vi "ConfigureElevator.vi"(10 "Talon In":T1) -> (2 "Talon Out":T1)   [LabVIEW 2018]
uses:
  <vilib>/Rock Robotics/WPI/MotorControl/WPI_MotorControlDeviceRef.ctl
  <vilib>/Rock Robotics/WPI/MotorControl/WPI_MotorControlType.ctl
  <vilib>/Rock Robotics/SystemInterfaces/DIO/FPGA_DIOPWMChannel.ctl
  <vilib>/Rock Robotics/WPI/PWM/WPI_PWMDeadband.ctl
  <vilib>/Rock Robotics/SystemInterfaces/DIO/FPGA_DIOChannel.ctl
  <vilib>/Rock Robotics/WPI/ThirdParty/Phoenix-LabVIEW/Motor Controller/Controls/CTRE_Phoenix_MotorControl_FeedbackDevice.ctl
  <vilib>/Rock Robotics/WPI/ThirdParty/Phoenix-LabVIEW/Motor Controller/Controls/CTRE_Phoenix_MotorControl_StatusFrameEnhanced.ctl
  <vilib>/Rock Robotics/WPI/ThirdParty/Phoenix-LabVIEW/Motor Controller/Controls/CTRE_Phoenix_MotorControl_NeutralMode.ctl
  <vilib>/Rock Robotics/WPI/ThirdParty/Phoenix-LabVIEW/Motor Controller/Controls/CTRE_Phoenix_MotorControl_ControlMode.ctl
  Elevator Constants.vi
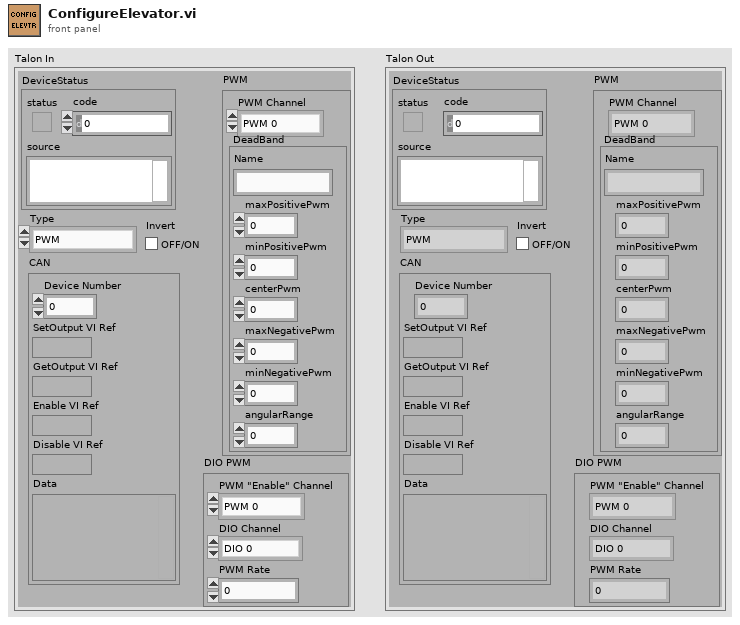
[diagram p1: front panel]
types:
  T1 = typedef "WPI_MotorControlDeviceRef.ctl" = cluster{"DeviceStatus":errorcluster, "Type":T2, "PWM":cluster{"PWM Channel":T3, "DeadBand":T4}, "CAN":cluster{"Device Number":u8, "SetOutput VI Ref":variant, "GetOutput VI Ref":variant, "Enable VI Ref":variant, "Disable VI Ref":variant, "Data":variant}, "Invert":bool, "DIO PWM":cluster{"PWM \"Enable\" Channel":T3, "DIOChannel":T5, "PWM Rate":dbl}}
  T2 = typedef "WPI_MotorControlType.ctl" = enum16{"PWM", "CAN", "DIO PWM"}
  T3 = typedef "FPGA_DIOPWMChannel.ctl" = enum8{"PWM 0", "PWM 1", "PWM 2", "PWM 3", "PWM 4", "PWM 5", "PWM 6", "PWM 7", "PWM 8", "PWM 9", "PWM MXP 0", "PWM MXP 1", "PWM MXP 2", "PWM MXP 3", "PWM MXP 4", "PWM MXP 5", "PWM MXP 6", "PWM MXP 7", "PWM MXP 8", "PWM MXP 9", "Invalid"}
  T4 = typedef "WPI_PWMDeadband.ctl" = cluster{"Name":string, "maxPositivePwm":i32, "minPositivePwm":i32, "centerPwm":i32, "maxNegativePwm":i32, "minNegativePwm":i32, "angularRange":u16}
  T5 = typedef "FPGA_DIOChannel.ctl" = enum8{"DIO 0", "DIO 1", "DIO 2", "DIO 3", "DIO 4", "DIO 5", "DIO 6", "DIO 7", "DIO 8", "DIO 9", "DIO MXP 0", "DIO MXP 1", "DIO MXP 2", "DIO MXP 3", "DIO MXP 4", "DIO MXP 5", "DIO MXP 6", "DIO MXP 7", "DIO MXP 8", "DIO MXP 9", "DIO MXP 10", "DIO MXP 11", "DIO MXP 12", "DIO MXP 13", "DIO MXP 14", "DIO MXP 15", "SPI Port CS1", "SPI Port CS2", "SPI Port CS3", "SPI Port MISO", "SPI Port MOSI", "Invalid"}
  T6 = typedef "CTRE_Phoenix_MotorControl_ControlMode.ctl" = u16
  T7 = typedef "CTRE_Phoenix_MotorControl_NeutralMode.ctl" = enum8{"EEPROMSetting", "Override to Coast", "Override to Brake"}
  T8 = typedef "CTRE_Phoenix_MotorControl_StatusFrameEnhanced.ctl" = u16
  T9 = typedef "CTRE_Phoenix_MotorControl_FeedbackDevice.ctl" = i8
  T10 = cluster{"kP":dbl, "kI ":dbl, "kD":dbl, "kF":dbl, "I Zone":dbl, "Peak Out":dbl}
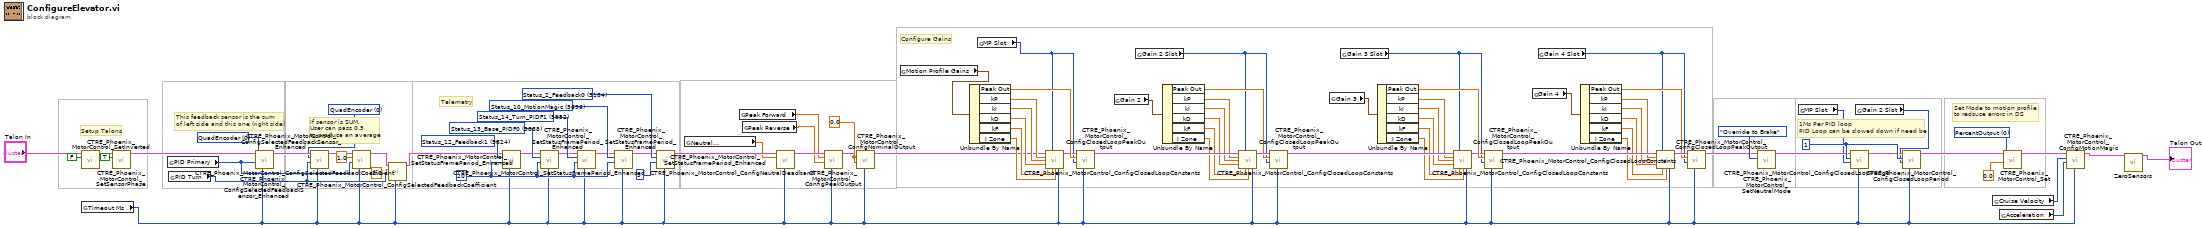
[diagram p0: block diagram]
diagram:
  w31 = T6 0 items=["PercentOutput"=0, "Position"=1, "Velocity"=2, "Current"=3, "Follower"=5, "MotionProfile"=6, "MotionMagic"=7, "MotionProfileArc"=10, "Disabled"=15] ("Control Mode")
  w89 = 1 ("loopTimeMs")
  w52 = 0.0 ("Forward Nominal Percent Output")
  w28 = 20 ("periodMs")
  w47 = T8 5184 items=["Status_1_General"=5120, "Status_2_Feedback0"=5184, "Status_3_Quadrature"=5248, "Status_4_AinTempVbat"=5312, "Status_6_Misc"=5440, "Status_7_CommStatus"=5504, "Status_8_PulseWidth"=5568, "Status_9_MotProfBuffer"=5632, "Status_10_MotionMagic"=5696, "Status_11_UartGadgeteer"=5760, "Status_12_Feedback1"=5824, "Status_13_Base_PIDF0"=5888, "Status_14_Turn_PIDF1"=5952, "Status_15_FirmwareApiStatus"=6016] ("Status Frame")
  w46 = T8 5696 items=["Status_1_General"=5120, "Status_2_Feedback0"=5184, "Status_3_Quadrature"=5248, "Status_4_AinTempVbat"=5312, "Status_6_Misc"=5440, "Status_7_CommStatus"=5504, "Status_8_PulseWidth"=5568, "Status_9_MotProfBuffer"=5632, "Status_10_MotionMagic"=5696, "Status_11_UartGadgeteer"=5760, "Status_12_Feedback1"=5824, "Status_13_Base_PIDF0"=5888, "Status_14_Turn_PIDF1"=5952, "Status_15_FirmwareApiStatus"=6016] ("Status Frame")
  w45 = T8 5952 items=["Status_1_General"=5120, "Status_2_Feedback0"=5184, "Status_3_Quadrature"=5248, "Status_4_AinTempVbat"=5312, "Status_6_Misc"=5440, "Status_7_CommStatus"=5504, "Status_8_PulseWidth"=5568, "Status_9_MotProfBuffer"=5632, "Status_10_MotionMagic"=5696, "Status_11_UartGadgeteer"=5760, "Status_12_Feedback1"=5824, "Status_13_Base_PIDF0"=5888, "Status_14_Turn_PIDF1"=5952, "Status_15_FirmwareApiStatus"=6016] ("Status Frame")
  w44 = T8 5888 items=["Status_1_General"=5120, "Status_2_Feedback0"=5184, "Status_3_Quadrature"=5248, "Status_4_AinTempVbat"=5312, "Status_6_Misc"=5440, "Status_7_CommStatus"=5504, "Status_8_PulseWidth"=5568, "Status_9_MotProfBuffer"=5632, "Status_10_MotionMagic"=5696, "Status_11_UartGadgeteer"=5760, "Status_12_Feedback1"=5824, "Status_13_Base_PIDF0"=5888, "Status_14_Turn_PIDF1"=5952, "Status_15_FirmwareApiStatus"=6016] ("Status Frame")
  w43 = T8 5824 items=["Status_1_General"=5120, "Status_2_Feedback0"=5184, "Status_3_Quadrature"=5248, "Status_4_AinTempVbat"=5312, "Status_6_Misc"=5440, "Status_7_CommStatus"=5504, "Status_8_PulseWidth"=5568, "Status_9_MotProfBuffer"=5632, "Status_10_MotionMagic"=5696, "Status_11_UartGadgeteer"=5760, "Status_12_Feedback1"=5824, "Status_13_Base_PIDF0"=5888, "Status_14_Turn_PIDF1"=5952, "Status_15_FirmwareApiStatus"=6016] ("Status Frame")
  w27 = T9 0 items=["None"=-1, "QuadEncoder"=0, "Analog"=2, "Tachometer"=4, "Pulse Width Encoded Position"=8, "Sensor Sum (S0 + S1)"=9, "Sensor Difference (D0 - D1)"=10, "Remote Source 0"=11, "Remote Source 1"=12, "Software Emulated"=15] ("Feedback Device")
  w35 = T9 0 items=["None"=-1, "QuadEncoder"=0, "Analog"=2, "Tachometer"=4, "Pulse Width Encoded Position"=8, "Sensor Sum (S0 + S1)"=9, "Sensor Difference (D0 - D1)"=10, "Remote Source 0"=11, "Remote Source 1"=12, "Software Emulated"=15] ("Feedback Device")
  # "Set Mode to motion profile\nto redsuce errors in DS"
  # "1Ms Per PID loop\nPID Loop can be slowed down if need be"
  # "Configure Gains"
  # "Setup Talons"
  # "Telemetry"
  # "If sensor is SUM,\nUser can pass 0.5\nto produce an average"
  # "This feedback sensor is the sum\nof left side and this one (right side)"
  n1 = call <vilib>:"CTRE_Phoenix_MotorControl_SetInverted.vi"("Invert?"=FALSE, "PhoenixMotorControlDevRef"="Talon In") -> ("PhoenixMotorControlDevRef"=w33:T1)  [unwired: 8 in, 1 out]
  n2 = global read "Elevator Constants.vi" "Timeout Ms"() -> (w2:i32)
  n3 = call <vilib>:"CTRE_Phoenix_MotorControl_SetSensorPhase.vi"("PhaseSensor"=TRUE, "PhoenixMotorControlDevRef"=w33) -> ("PhoenixMotorControlDevRef"=w24:T1)  [unwired: 8 in, 1 out]
  n4 = global read "Elevator Constants.vi" "PID Primary"() -> (w22:i32)
  n5 = global read "Elevator Constants.vi" "PID Turn"() -> (w21:i32)
  n6 = call <vilib>:"CTRE_Phoenix_MotorControl_ConfigSelectedFeedbackSensor_Enhanced.vi"("timeoutMs"=w2, "pidLoopIdx"=w22, "Feedback Device"=w35, "PhoenixMotorControlDevRef"=w24) -> ("PhoenixMotorControlDevRef"=w36:T1)  [unwired: 6 in, 1 out]
  n7 = call <vilib>:"CTRE_Phoenix_MotorControl_ConfigSelectedFeedbackSensor_Enhanced.vi"("timeoutMs"=w2, "pidLoopIdx"=w21, "Feedback Device"=w27, "PhoenixMotorControlDevRef"=w36) -> ("PhoenixMotorControlDevRef"=w37:T1)  [unwired: 6 in, 1 out]
  n8 = call <vilib>:"CTRE_Phoenix_MotorControl_ConfigSelectedFeedbackCoefficient.vi"("timoutMs"=w2, "pidIdx"=w22, "coefficient"=1.0, "PhoenixMotorControlDevRef"=w37) -> ("PhoenixMotorControlDevRef"=w26:T1)  [unwired: 6 in, 1 out]
  n9 = call <vilib>:"CTRE_Phoenix_MotorControl_ConfigSelectedFeedbackCoefficient.vi"("timoutMs"=w2, "pidIdx"=w21, "coefficient"=1.0, "PhoenixMotorControlDevRef"=w26) -> ("PhoenixMotorControlDevRef"=w25:T1)  [unwired: 6 in, 1 out]
  n10 = call <vilib>:"CTRE_Phoenix_MotorControl_SetStatusFramePeriod_Enhanced.vi"("timeoutMs"=w2, "periodMs"=w28, "Status Frame"=w43, "PhoenixMotorControlDevRef"=w25) -> ("PhoenixMotorControlDevRef"=w39:T1)  [unwired: 6 in, 1 out]
  n11 = call <vilib>:"CTRE_Phoenix_MotorControl_SetStatusFramePeriod_Enhanced.vi"("timeoutMs"=w2, "periodMs"=w28, "Status Frame"=w44, "PhoenixMotorControlDevRef"=w39) -> ("PhoenixMotorControlDevRef"=w40:T1)  [unwired: 6 in, 1 out]
  n12 = call <vilib>:"CTRE_Phoenix_MotorControl_SetStatusFramePeriod_Enhanced.vi"("timeoutMs"=w2, "periodMs"=w28, "Status Frame"=w45, "PhoenixMotorControlDevRef"=w40) -> ("PhoenixMotorControlDevRef"=w41:T1)  [unwired: 6 in, 1 out]
  n13 = call <vilib>:"CTRE_Phoenix_MotorControl_SetStatusFramePeriod_Enhanced.vi"("timeoutMs"=w2, "periodMs"=w28, "Status Frame"=w46, "PhoenixMotorControlDevRef"=w41) -> ("PhoenixMotorControlDevRef"=w42:T1)  [unwired: 6 in, 1 out]
  n14 = call <vilib>:"CTRE_Phoenix_MotorControl_SetStatusFramePeriod_Enhanced.vi"("timeoutMs"=w2, "periodMs"=5, "Status Frame"=w47, "PhoenixMotorControlDevRef"=w42) -> ("PhoenixMotorControlDevRef"=w49:T1)  [unwired: 6 in, 1 out]
  n15 = global read "Elevator Constants.vi" "Neutral\nDeadband"() -> (w20:dbl)
  n16 = global read "Elevator Constants.vi" "Peak Forward"() -> (w6:dbl)
  n17 = global read "Elevator Constants.vi" "Peak Reverse"() -> (w7:dbl)
  n18 = call <vilib>:"CTRE_Phoenix_MotorControl_ConfigNeutralDeadband.vi"("timeoutMs"=w2, "Percent Deadband"=w20, "PhoenixMotorControlDevRef"=w49) -> ("PhoenixMotorControlDevRef"=w50:T1)  [unwired: 7 in, 1 out]
  n19 = call <vilib>:"CTRE_Phoenix_MotorControl_ConfigPeakOutput.vi"("timeoutMs"=w2, "Reverse Peak Percent Output"=w7, "Forward Peak Percent Output"=w6, "PhoenixMotorControlDevRef"=w50) -> ("PhoenixMotorControlDevRef"=w51:T1)  [unwired: 6 in, 1 out]
  n20 = call <vilib>:"CTRE_Phoenix_MotorControl_ConfigNominalOutput.vi"("timeoutMs"=w2, "Reverse Nominal Percent Output"=w52, "Forward Nominal Percent Output"=w52, "PhoenixMotorControlDevRef"=w51) -> ("PhoenixMotorControlDevRef"=w53:T1)  [unwired: 6 in, 1 out]
  n21 = global read "Elevator Constants.vi" "Motion Profile Gains"() -> (w19:T10)
  n22 = Unbundle By Name(w19) -> ("Peak Out"=w60:dbl, "kP"=w54:dbl, "kI"=w55:dbl, "kD"=w56:dbl, "kF"=w57:dbl, "I Zone"=w58:dbl)
  n23 = global read "Elevator Constants.vi" "MP Slot"() -> (w17:i32)
  n24 = call <vilib>:"CTRE_Phoenix_MotorControl_ConfigClosedLoopConstants.vi"("PhoenixMotorControlDevRef"=w53, "slotIdx"=w17, "P"=w54, "I"=w55, "D"=w56, "F"=w57, "I Zone"=w58, "timeoutMs"=w2) -> ("PhoenixMotorControlDevRef"=w59:T1)  [unwired: 6 in, 1 out]
  n25 = call <vilib>:"CTRE_Phoenix_MotorControl_ConfigClosedLoopPeakOutput.vi"("timoutMs"=w2, "slotIdx"=w17, "peakOutput"=w60, "PhoenixMotorControlDevRef"=w59) -> ("PhoenixMotorControlDevRef"=w82:T1)  [unwired: 6 in, 1 out]
  n26 = global read "Elevator Constants.vi" "Gain 2"() -> (w18:T10)
  n27 = global read "Elevator Constants.vi" "Gain 2 Slot"() -> (w16:i32)
  n28 = Unbundle By Name(w18) -> ("Peak Out"=w61:dbl, "kP"=w67:dbl, "kI"=w66:dbl, "kD"=w65:dbl, "kF"=w64:dbl, "I Zone"=w63:dbl)
  n29 = call <vilib>:"CTRE_Phoenix_MotorControl_ConfigClosedLoopConstants.vi"("PhoenixMotorControlDevRef"=w82, "slotIdx"=w16, "P"=w67, "I"=w66, "D"=w65, "F"=w64, "I Zone"=w63, "timeoutMs"=w2) -> ("PhoenixMotorControlDevRef"=w62:T1)  [unwired: 6 in, 1 out]
  n30 = call <vilib>:"CTRE_Phoenix_MotorControl_ConfigClosedLoopPeakOutput.vi"("timoutMs"=w2, "slotIdx"=w16, "peakOutput"=w61, "PhoenixMotorControlDevRef"=w62) -> ("PhoenixMotorControlDevRef"=w83:T1)  [unwired: 6 in, 1 out]
  n31 = global read "Elevator Constants.vi" "Gain 3"() -> (w15:T10)
  n32 = global read "Elevator Constants.vi" "Gain 3 Slot"() -> (w14:i32)
  n33 = Unbundle By Name(w15) -> ("Peak Out"=w74:dbl, "kP"=w68:dbl, "kI"=w69:dbl, "kD"=w70:dbl, "kF"=w71:dbl, "I Zone"=w72:dbl)
  n34 = call <vilib>:"CTRE_Phoenix_MotorControl_ConfigClosedLoopConstants.vi"("PhoenixMotorControlDevRef"=w83, "slotIdx"=w14, "P"=w68, "I"=w69, "D"=w70, "F"=w71, "I Zone"=w72, "timeoutMs"=w2) -> ("PhoenixMotorControlDevRef"=w73:T1)  [unwired: 6 in, 1 out]
  n35 = call <vilib>:"CTRE_Phoenix_MotorControl_ConfigClosedLoopPeakOutput.vi"("timoutMs"=w2, "slotIdx"=w14, "peakOutput"=w74, "PhoenixMotorControlDevRef"=w73) -> ("PhoenixMotorControlDevRef"=w84:T1)  [unwired: 6 in, 1 out]
  n36 = global read "Elevator Constants.vi" "Gain 4"() -> (w13:T10)
  n37 = global read "Elevator Constants.vi" "Gain 4 Slot"() -> (w12:i32)
  n38 = Unbundle By Name(w13) -> ("Peak Out"=w75:dbl, "kP"=w81:dbl, "kI"=w80:dbl, "kD"=w79:dbl, "kF"=w78:dbl, "I Zone"=w77:dbl)
  n39 = call <vilib>:"CTRE_Phoenix_MotorControl_ConfigClosedLoopConstants.vi"("PhoenixMotorControlDevRef"=w84, "slotIdx"=w12, "P"=w81, "I"=w80, "D"=w79, "F"=w78, "I Zone"=w77, "timeoutMs"=w2) -> ("PhoenixMotorControlDevRef"=w76:T1)  [unwired: 6 in, 1 out]
  n40 = call <vilib>:"CTRE_Phoenix_MotorControl_ConfigClosedLoopPeakOutput.vi"("timoutMs"=w2, "slotIdx"=w12, "peakOutput"=w75, "PhoenixMotorControlDevRef"=w76) -> ("PhoenixMotorControlDevRef"=w85:T1)  [unwired: 6 in, 1 out]
  n41 = call <vilib>:"CTRE_Phoenix_MotorControl_SetNeutralMode.vi"("Motor Control Neutral Mode"=CTRE_Phoenix_MotorControl_NeutralMode."Override to Brake", "PhoenixMotorControlDevRef"=w85) -> ("PhoenixMotorControlDevRef"=w87:T1)  [unwired: 8 in, 1 out]
  n42 = global read "Elevator Constants.vi" "MP Slot"() -> (w11:i32)
  n43 = call <vilib>:"CTRE_Phoenix_MotorControl_ConfigClosedLoopPeriod.vi"("timoutMs"=w2, "slotIdx"=w11, "loopTimeMs"=w89, "PhoenixMotorControlDevRef"=w87) -> ("PhoenixMotorControlDevRef"=w88:T1)  [unwired: 6 in, 1 out]
  n44 = global read "Elevator Constants.vi" "Gain 2 Slot"() -> (w10:i32)
  n45 = call <vilib>:"CTRE_Phoenix_MotorControl_ConfigClosedLoopPeriod.vi"("timoutMs"=w2, "slotIdx"=w10, "loopTimeMs"=w89, "PhoenixMotorControlDevRef"=w88) -> ("PhoenixMotorControlDevRef"=w9:T1)  [unwired: 6 in, 1 out]
  n46 = global read "Elevator Constants.vi" "Cruise Velocity"() -> (w4:i32)
  n47 = global read "Elevator Constants.vi" "Acceleration"() -> (w3:i32)
  n48 = call <vilib>:"CTRE_Phoenix_MotorControl_Set.vi"("Output"=0.0, "Control Mode"=w31, "PhoenixMotorControlDevRef"=w9) -> ("PhoenixMotorControlDevRef"=w5:T1)  [unwired: 7 in, 1 out]
  n49 = call <vilib>:"CTRE_Phoenix_MotorControl_ConfigMotionMagic.vi"("timeoutMs"=w2, "Acceleration"=w3, "Cruise Velocity"=w4, "PhoenixMotorControlDevRef"=w5) -> ("PhoenixMotorControlDevRef"=w1:T1)  [unwired: 6 in, 1 out]
  n50 = call "ZeroSensors.vi"("Talon 1"=w1) -> ("Talon 1"=→"Talon Out":T1)  [unwired: 8 in, 2 out]
